vi "Servo Close N Channels.vi"(8 "Error In":errorcluster, 10 "Servo Channels":u8[](array[numeric]), 11 "LINX Resource":T1) -> (0 "Error Out":errorcluster, 3 "LINX Resource":T1)   [LabVIEW 2014, in "LMH-LINX.lvlib" / "Servo.lvlib"]
doc: "Read the values of the specified digital input channels."
uses:
  <vilib>/MakerHub/LINX/Public/Sensors/Motion/Servo/Servo.lvlib
  <vilib>/MakerHub/LINX/Private/Type Defs/LINX Ref.ctl
  <vilib>/MakerHub/LINX/Private/Type Defs/Platform.ctl
  <vilib>/MakerHub/LINX/Private/Type Defs/Interface.ctl
  <vilib>/MakerHub/LINX/Private/Device/Type Defs/LINX Device Config.ctl
  <vilib>/MakerHub/LINX/Private/Device/Type Defs/TCP Config.ctl
  <vilib>/MakerHub/LINX/Private/Device/Type Defs/Channels.ctl
  <vilib>/MakerHub/LINX/Private/Type Defs/Peripheral.ctl
  <vilib>/MakerHub/LINX/Private/Type Defs/Error Type.ctl
  <vilib>/MakerHub/LINX/LMH-LINX.lvlib
  <vilib>/MakerHub/LINX/Private/Device/Device.lvlib
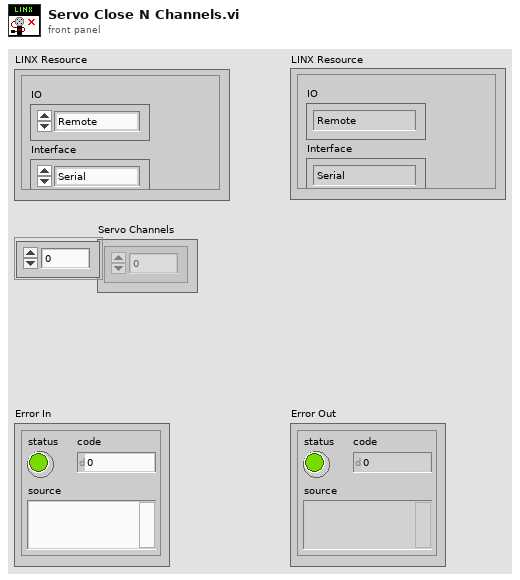
[diagram p1: front panel]
types:
  T1 = typedef "LMH-LINX.lvlib/LINX Ref.ctl" = cluster{"IO":T2, "Interface":T3, "LINX Device Config":T4}
  T2 = typedef "LMH-LINX.lvlib/Platform.ctl" = enum16{"Remote", "Local"}
  T3 = typedef "LMH-LINX.lvlib/Interface.ctl" = enum16{"Serial", "TCP"}
  T4 = typedef "LMH-LINX.lvlib/Device.lvlib/LINX Device Config.ctl" = cluster{"Interface":T3, "COM Port":refnum<visa-resource-name>, "TCP Configuration":T5, "Device Family":u8, "Device ID":u8, "Device Name":string, "TCP Ref":refnum<k5>, "Channels":T6}
  T5 = typedef "LMH-LINX.lvlib/Device.lvlib/TCP Config.ctl" = cluster{"IP Address":string, "Port":u16}
  T6 = typedef "LMH-LINX.lvlib/Channels.ctl" = cluster{"DI":u8[], "DO":u8[], "AI":u8[], "AO":u8[], "PWM":u8[], "QE":u8[], "UART":u8[], "I2C 2":u8[], "SPI":u8[], "CAN":u8[], "Servo":u8[], "AI Ref (V)":dbl, "AI Resolution (Bits)":u8, "AO Ref (V)":dbl, "AO Resolution (Bits)":u8}
  T7 = typedef "LMH-LINX.lvlib/Peripheral.ctl" = enum8{"DI", "DO", "AI", "AO", "PWM", "QE", "UART", "I2C", "SPI", "CAN", "Servo"}
  T8 = typedef "LMH-LINX.lvlib/Error Type.ctl" = enum16{"Unknown", "Timeout", "Corrupt Return Packet", "Unable To Connect", "Command Not Supported", "Channel DNE", "Invalid COM Config", "Firmware Version Mismatch", "myRIO Support", "CMD Specific Error", "Local IO Not Supported"}
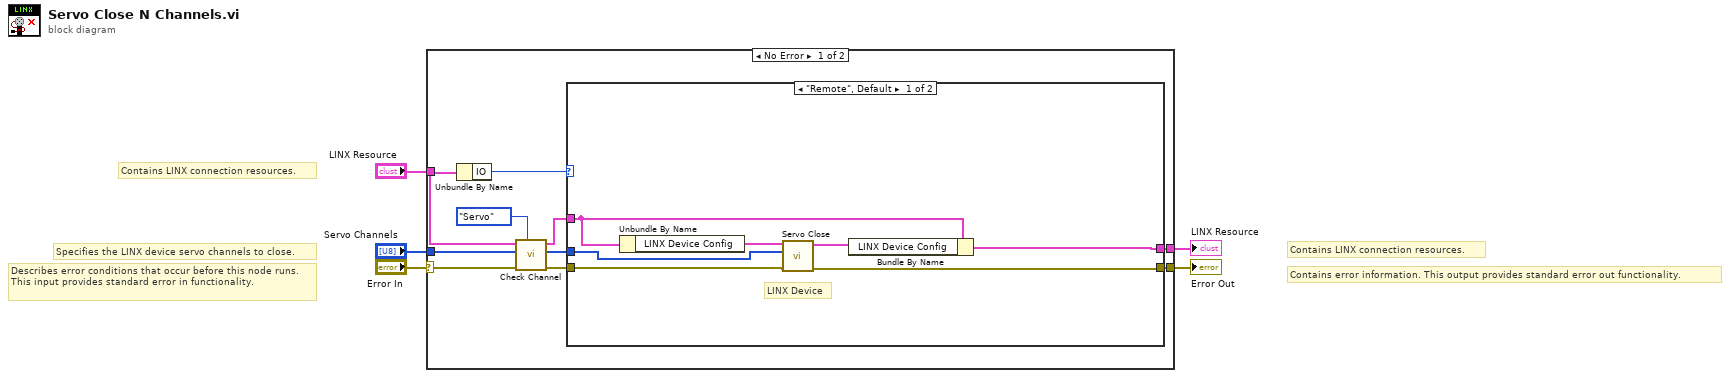
[diagram p0: block diagram]
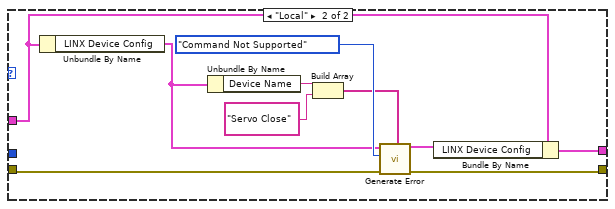
[diagram p2: hidden frame]
diagram:
  # "Specifies the LINX device servo channels to close."
  # "Contains LINX connection resources."
  # "Contains error information. This output provides standard error out functionality."
  # "Contains LINX connection resources."
  # "Describes error conditions that occur before this node runs. This input provides standard error in functionality."
  n1 = case shown="No Error" "Error In" {
    selector: "Error In" -> [w6 w34]
    tunnel: [w14 w34] -> w5
    tunnel: [w13 w33] -> w4
    tunnel: "LINX Resource" -> [w8 w33]
    tunnel: "Servo Channels" -> [w7 _]
    frame No Error {
      n2 = Unbundle By Name(w8) -> ("IO"=w15:T2)
      n3 = call <vilib>:"Check Channel.vi"("Peripheral"=Peripheral."Servo", "Error In"=w6, "Channels"=w7, "LINX Resource"=w8) -> ("Error Out"=w12:errorcluster, "Channels"=w11:u8[], "LINX Resource"=w9:T1)  [unwired: 5 in]
      n4 = case shown="\"Remote\", Default" w15 {
        tunnel: w12 -> [w20 w32]
        tunnel: w9 -> [w22 w25]
        tunnel: [w19 w31] -> w14
        tunnel: [w21 w23] -> w13
        tunnel: w11 -> [w18 _]
        frame "Remote", Default {
          # "LINX Device"
          n5 = Unbundle By Name(w22) -> ("LINX Device Config"=w16:T4)
          n6 = call <vilib>:"Servo Close.vi"("Error In"=w20, "Channels"=w18, "LINX Device Config"=w16) -> ("Error Out"=w19:errorcluster, "LINX Device Config"=w17:T4)  [unwired: 7 in]
          n7 = Bundle By Name(cluster=w22, "LINX Device Config"=w17) -> (w21:T1)
        }
        frame "Local" {
          n8 = Unbundle By Name(w25) -> ("LINX Device Config"=w26:T4)
          n9 = Unbundle By Name(w26) -> ("Device Name"=w30:string)
          n10 = Build Array(w30, "Servo Close") -> (w27:string[])
          n11 = call <vilib>:"Generate Error.vi"("Error In"=w32, "Arguments"=w27, "Error Type"=Error_Type."Command Not Supported", "LINX Device Config"=w26) -> ("Error Out"=w31:errorcluster, "Dup LINX Device Config"=w24:T4)  [unwired: 6 in]
          n12 = Bundle By Name(cluster=w25, "LINX Device Config"=w24) -> (w23:T1)
        }
      }
    }
    frame Error {
    }
  }
  "Error Out" <- w5
  "LINX Resource" <- w4
